vi "Finalize.vi"(8 "error in":errorcluster, 11 "Log Producer in":refnum<class "Log Producer.lvclass">) -> (0 "error out":errorcluster, 2 "Logger":refnum<class "Logger Interface.lvclass">, 3 "Log Producer out":refnum<class "Log Producer.lvclass">)   [LabVIEW 2020, in "AIM ARINC 664 Engine.lvlib" / "Implementation.lvlib" / "Frame Logging.lvlib" / "Log Producer.lvclass"]
uses:
  Log Producer.lvclass
  Logger Interface/Logger Interface.lvclass
  Log Producer.lvclass/Log Producer.ctl
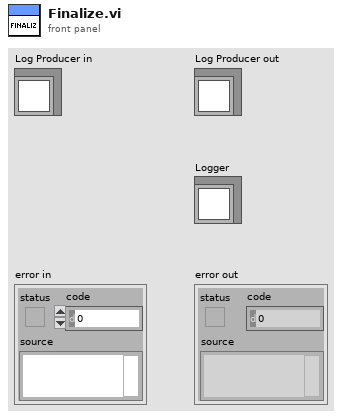
[diagram p1: front panel]
types:
  T1 = typedef "AIM ARINC 664 Engine.lvlib/Implementation.lvlib/Frame Logging.lvlib/Logger Data Reference.ctl" = refnum<data-value>
  T2 = cluster{"Logger Interface.lvclass":refnum<class "Logger Interface.lvclass">}
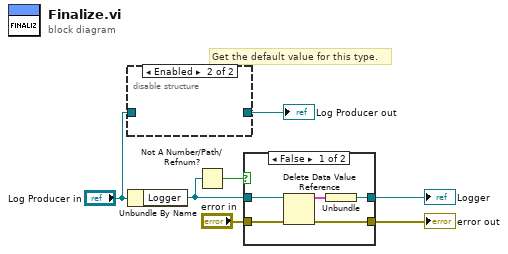
[diagram p0: block diagram]
diagram:
  # "Get the default value for this type."
  n1 = disable-structure shown="Enabled" {
    disable-tunnel: "Log Producer in" -> [w8 _]
    disable-tunnel: [w8 _] -> w4
    frame Disabled {
    }
    frame Enabled {
    }
  }
  "Log Producer out" <- w4
  n2 = Unbundle By Name("Log Producer in") -> ("Logger"=w7:T1)
  n3 = Not A Number/Path/Refnum?(number/path/refnum=w7) -> (NaN/Path/Refnum?=w6:bool)
  n4 = case shown="False" w6 {
    tunnel: [w11 w14] -> w2
    tunnel: "error in" -> [w13 w14]
    tunnel: w7 -> [w12 _]
    tunnel: [w9 _] -> w1
    frame False {
      n5 = Delete Data Value Reference(data value reference=w12, error in=w13) -> (data value=w10:T2, error out=w11:errorcluster)
      n6 = Unbundle(w10) -> ("Logger Interface.lvclass"=w9:refnum<class "Logger Interface.lvclass">)
    }
    frame True {
    }
  }
  "error out" <- w2
  "Logger" <- w1
